vi "ComplementNB.vi"(8 "error in":errorcluster) -> (0 "error out":errorcluster, 3 "out":refnum<class "ComplementNB.lvclass">)   [LabVIEW 2020]
doc: "The Complement Naive Bayes classifier described in Rennie et al. (2003).\n\n The Complement Naive Bayes classifier was designed to correct the \"severe\n assumptions\" made by the standard Multinomial Naive Bayes classifier. It is\n particularly suited for imbalanced data sets.\n\n Read more in the :ref:`User Guide <complement_naive_bayes>`.\n\n .. versionadded:: 0.20\n\n Parameters\n ----------\n alpha : float, default=1.0\n Additive (Laplace/Lidstone) smoothing parameter (0 for no smoothing).\n\n fit_prior : bool, default=True\n Only used in edge case with a single class in the training set.\n\n class_prior : array-like of shape (n_classes,), default=None\n Prior probabilities of the classes. Not used.\n\n norm : bool, default=False\n Whether or not a second normalization of the weights is performed. The\n default behavior mirrors the implementations found in Mahout and Weka,\n which do not follow the full algorithm described in Table 9 of the\n paper.\n\n Attributes\n ----------\n class_count_ : ndarray of shape (n_classes,)\n Number of samples encountered for each class during fitting. This\n value is weighted by the sample weight when provided.\n\n class_log_prior_ : ndarray of shape (n_classes,)\n Smoothed empirical log probability for each class. Only used in edge\n case with a single class in the training set.\n\n classes_ : ndarray of shape (n_classes,)\n Class labels known to the classifier\n\n coef_ : ndarray of shape (n_classes, n_features)\n Mirrors ``feature_log_prob_`` for interpreting `ComplementNB`\n as a linear model.\n\n .. deprecated:: 0.24\n ``coef_`` is deprecated in 0.24 and will be removed in 1.1\n (renaming of 0.26).\n\n feature_all_ : ndarray of shape (n_features,)\n Number of samples encountered for each feature during fitting. This\n value is weighted by the sample weight when provided.\n\n feature_count_ : ndarray of shape (n_classes, n_features)\n Number of samples encountered for each (class, feature) during fitting.\n This value is weighted by the sample weight when provided.\n\n feature_log_prob_ : ndarray of shape (n_classes, n_features)\n Empirical weights for class complements.\n\n intercept_ : ndarray of shape (n_classes,)\n Mirrors ``class_log_prior_`` for interpreting `ComplementNB`\n as a linear model.\n\n .. deprecated:: 0.24\n ``coef_`` is deprecated in 0.24 and will be removed in 1.1\n (renaming of 0.26).\n\n n_features_ : int\n Number of features of each sample.\n\n \nAvailable methods:\nFit\nPartial Fit\nPredict\nPredict Log Proba\nPredict Proba\nScore\nGet Attributes\nGet Params\nSet Params"
uses:
  ComplementNB.lvclass
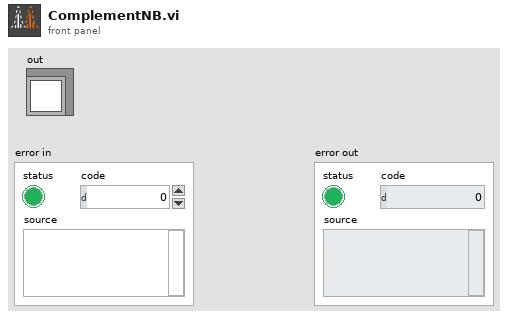
[diagram p1: front panel]
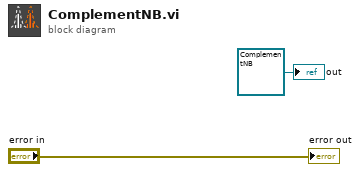
[diagram p0: block diagram]
diagram:
  "out" <- refnum<class "ComplementNB.lvclass"> refnum ("model")
  "error out" <- "error in"
